vi "FT_Read_Byte_Data.vi"(8 "error in (no error)":errorcluster, 10 "Bytes To Read":u32, 11 "Handle In":u64) -> (0 "error out":errorcluster, 1 "FT_Status":u32(ring) items=["FT_OK", "FT_INVALID_HANDLE", "FT_DEVICE_NOT_FOUND", "FT_DEVICE_NOT_OPENED", "FT_IO_ERROR", "FT_INSUFFICIENT_RESOURCES", "FT_INVALID_PARAMETER", "FT_INVALID_BAUD_RATE", "FT_DEVICE_NOT_OPENED_FOR_ERASE", "FT_DEVICE_NOT_OPENED_FOR_WRITE", "FT_FAILED_TO_WRITE_DEVICE", "FT_EEPROM_READ_FAILED", "FT_EEPROM_WRITE_FAILED", "FT_EEPROM_ERASE_FAILED", "FT_EEPROM_NOT_PRESENT", "FT_EEPROM_NOT_PROGRAMMED", "FT_INVALID_ARGS", "FT_NOT_SUPPORTED", "FT_OTHER_ERROR"], 2 "Read Data":u8[](array[numeric]), 3 "Handle Out":u64, 4 "Bytes Read":u32)   [LabVIEW 2018]
uses:
  FTD2XX.dll
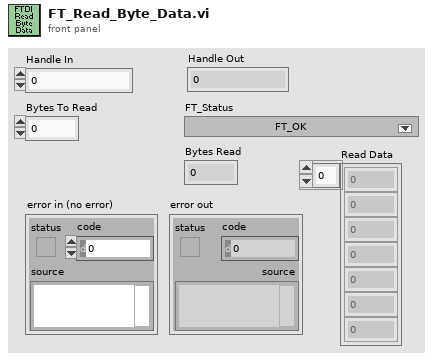
[diagram p1: front panel]
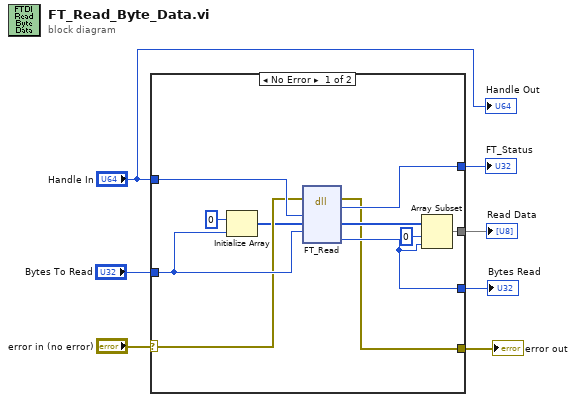
[diagram p0: block diagram]
diagram:
  n1 = case shown="No Error" "error in (no error)" {
    selector: "error in (no error)" -> [w9 w19]
    tunnel: [w18 _] -> w7
    tunnel: "Bytes To Read" -> [w17 _]
    tunnel: [w13 _] -> w5
    tunnel: [w12 _] -> w4
    tunnel: "Handle In" -> [w11 _]
    tunnel: [w10 w19] -> w3
    frame No Error {
      n2 = Initialize Array(u8 0 ("element"), w17) -> (w8:u8[])
      n3 = dll-call lib="FTD2XX.dll" fn="FT_Read"(error in=w9, "Handle"=w11, "Buffer"=w8, "BytesToRead"=w17) -> (error out=w10:errorcluster, "FT_Status"=w18:u32, "Buffer"=w15:u8[], "BytesReturned"=w13:u32)  [unwired: 5 in, 1 out]
      n4 = Array Subset(array=w15, index=0, length=w13) -> (w12:u8[])
    }
    frame Error {
    }
  }
  "FT_Status" <- w7
  "Bytes Read" <- w5
  "Read Data" <- w4
  "error out" <- w3
  "Handle Out" <- "Handle In"
